vi "_Init ActiveUIRef.vi"(8 "error in (no error)":errorcluster, 11 "UI_ProgressDlg in":refnum<class "UI_ProgressDlg.lvclass">) -> (0 "error out":errorcluster, 3 "UI_ProgressDlg out":refnum<class "UI_ProgressDlg.lvclass">)   [LabVIEW 2014, in "UI_ProgressDlg.lvlib" / "UI_ProgressDlg.lvclass"]
uses:
  UI_ProgressDlg.lvclass
  UI_ProgressDlg.lvclass/UI_ProgressDlg.ctl
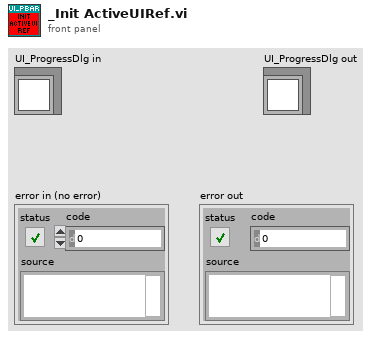
[diagram p1: front panel]
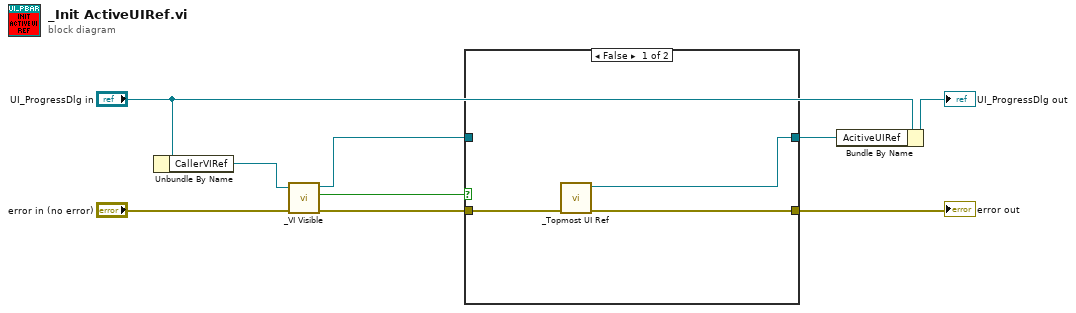
[diagram p0: block diagram]
diagram:
  n1 = Unbundle By Name("UI_ProgressDlg in") -> ("CallerVIRef"=w6:refnum<vi>)
  n2 = call "_VI Visible.vi"("error in (no error)"="error in (no error)", "VI in"=w6) -> ("error out"=w8:errorcluster, "visible"=w3:bool, "VI out"=w1:refnum<vi>)  [unwired: 7 in]
  n3 = case shown="False" w3 {
    tunnel: w8 -> [w12 w13]
    tunnel: [w10 w13] -> w4
    tunnel: [w11 w14] -> w2
    tunnel: w1 -> [_ w14]
    frame False {
      n4 = call "_Topmost UI Ref.vi"("error in (no error)"=w12) -> ("error out"=w10:errorcluster, "VI out"=w11:refnum<vi>)  [unwired: 9 in]
    }
    frame True {
    }
  }
  "error out" <- w4
  n5 = Bundle By Name(cluster="UI_ProgressDlg in", "AcitiveUIRef"=w2) -> (→"UI_ProgressDlg out":refnum<class "UI_ProgressDlg.lvclass">)
